vi "CosineBasedAccelerationControlOneMotor.vi"(0 "Target":dbl, 1 "Current Output":dbl, 2 "Loop Count":dbl, 3 "Acceleration Scaling Constant":dbl) -> (5 "Output":dbl)   [LabVIEW 2014]
panel:
  out "Target - Current":dbl
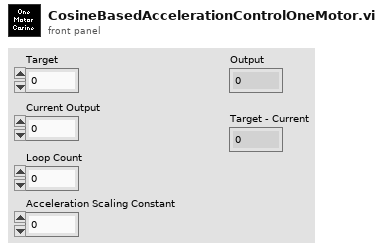
[diagram p1: front panel]
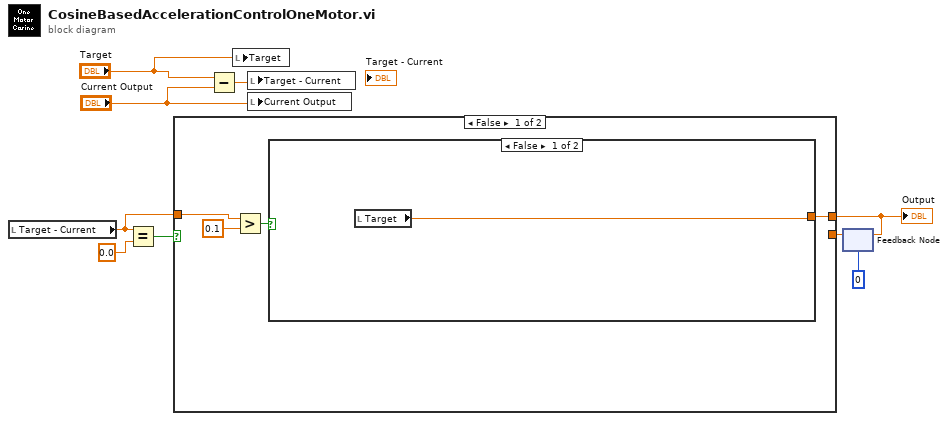
[diagram p0: block diagram]
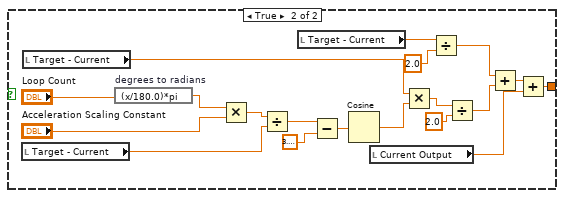
[diagram p2: hidden frame]
diagram:
  n1 = local read "Target - Current"() -> (w2:dbl)
  n2 = Equal?(x=w2, y=0.0) -> (x = y?=w6:bool)
  n3 = Subtract(x="Target", y="Current Output") -> (x-y=w9:dbl)
  n4 = local write "Target"("Target") -> ()
  n5 = local write "Target - Current"(w9) -> ()
  n6 = local write "Current Output"("Current Output") -> ()
  n7 = feedback #1(0) -> (w5:dbl)
  n8 = case shown="False" w6 {
    tunnel: w5 -> [_ w34]
    tunnel: [w13 w34] -> w3
    tunnel: w2 -> [w10 _]
    frame False {
      n9 = Greater?(x=w10, y=0.1) -> (0:w12:bool)
      n10 = case shown="False" w12 {
        tunnel: [w14 w15] -> w13
        frame False {
          n11 = local read "Target"() -> (w14:dbl)
        }
        frame True {
          n12 = local read "Target - Current"() -> (w16:dbl)
          n13 = local read "Target - Current"() -> (w25:dbl)
          n14 = expression code="(x/180.0)*pi" "degrees to radians"("Loop Count") -> (w18:dbl)
          n15 = Multiply(x=w18, y="Acceleration Scaling Constant") -> (x*y=w20:dbl)
          n16 = Divide(x=w20, y=w16) -> (x/y=w21:dbl)
          n17 = local read "Target - Current"() -> (w30:dbl)
          n18 = Subtract(x=w21, y=3.141592653589793) -> (x-y=w23:dbl)
          n19 = Cosine(x=w23) -> (cos(x)=w24:dbl)
          n20 = local read "Current Output"() -> (w33:dbl)
          n21 = Multiply(x=w25, y=w24) -> (x*y=w26:dbl)
          n22 = Divide(x=w30, y=2.0) -> (x/y=w31:dbl)
          n23 = Divide(x=w26, y=2.0) -> (x/y=w28:dbl)
          n24 = Add(x=w31, y=w28) -> (x+y=w32:dbl)
          n25 = Add(x=w32, y=w33) -> (x+y=w15:dbl)
        }
      }
    }
    frame True {
    }
  }
  "Output" <- w3
  n26 = feedback-in #1(w3) -> ()
